vi "Dispatch Shutdown.vi"(8 "error in (no error)":errorcluster, 11 "Dispatcher in":refnum<class "Dispatcher Thread.lvclass">) -> (0 "error out":errorcluster, 3 "Dispatcher out":refnum<class "Dispatcher Thread.lvclass">)   [LabVIEW 2021, in "DSF Core.lvlib" / "Dispatcher Thread.lvclass"]
uses:
  Dispatcher Thread.lvclass
  C:/dev/git/custom-devices/niveristand-data-sharing-framework-custom-device/Source/Core/Classes/Thread/Thread.lvclass
  Dispatcher Thread.lvclass/Dispatcher Thread.ctl
  Interface/Dispatcher/Response Data.ctl
  Interface/Dispatcher/Response.ctl
  Interface/Dispatcher/Parameters.ctl
  Thread.lvclass/Thread.ctl
  <vilib>/NI/Memory Manager/Classes/Pointer/Pointer.lvclass/Pointer.ctl
  <vilib>/NI/Memory Manager/Classes/Pointer/Write Bool.vi
  <vilib>/NI/Memory Manager/Classes/Pointer/Write (No Check).vi
  <vilib>/NI/Memory Manager/Classes/Pointer/Write (No Check) Bool.vi
  <vilib>/NI/Memory Manager/Classes/Pointer/Check Move.vi
  <vilib>/NI/Memory Manager/Classes/Pointer/Get Address.vi
  <vilib>/NI/Memory Manager/Classes/Pointer/Check Null Pointer.vi
  <vilib>/NI/Memory Manager/Classes/Pointer/Check Count.vi
  <vilib>/NI/Memory Manager/Classes/Pointer/Check Bounds (Power of 2).vi
  <vilib>/NI/Memory Manager/Classes/Pointer/Errors.vi
  <vilib>/NI/Memory Manager/Classes/Pointer/Null Pointer.vi
  <vilib>/NI/Memory Manager/Classes/Pointer/Is Null.vi
  <vilib>/NI/Memory Manager/Classes/Pointer/Get Size.vi
  <vilib>/NI/Memory Manager/Classes/Pointer/Out of Bounds.vi
  <vilib>/NI/Memory Manager/Classes/Pointer/Check Bounds.vi
  <vilib>/NI/Memory Manager/Classes/Pointer/Create Error.vi
  <vilib>/NI/Memory Manager/VIs/Write String to Source.vi
  <vilib>/NI/Memory Manager/Classes/Pointer/Write Pointer Size to Error.vi
  <vilib>/NI/Memory Manager/VIs/Write Numeric to Source.vi
  <vilib>/NI/Memory Manager/VIs/Write Numeric Scalar to Source (Base10 U64).vi
  <vilib>/NI/Memory Manager/Classes/Pointer/Check Bounds (Pointer).vi
  <vilib>/NI/Memory Manager/Classes/Pointer/Check Bounds (Buffer).vi
  <vilib>/NI/Memory Manager/VIs/New Error Cluster.vi
  <vilib>/NI/Memory Manager/VIs/New Error Cluster (512B).vi
  <vilib>/NI/Memory Manager/VIs/Set Error Status.vi
  <vilib>/NI/Memory Manager/VIs/Set Error Code.vi
  <vilib>/NI/Memory Manager/VIs/Set Error Source.vi
  <vilib>/NI/Memory Manager/Constants/Constants.vi
  <vilib>/NI/Memory Manager/Constants/Library Name.vi
  <vilib>/NI/Memory Manager/Classes/Pointer/Pointer Error Info.vi
  <vilib>/NI/Memory Manager/Constants/Pointer Class Name.vi
  <vilib>/NI/Memory Manager/Classes/Pointer/Buffer Underflow.vi
  Interface/Dispatcher/Write Dispatcher Response.vi
  Interface/Plugin/Plugin Interface.lvclass
  Thread.lvclass
  Interface/Dispatcher/Dispatcher Interface.lvclass
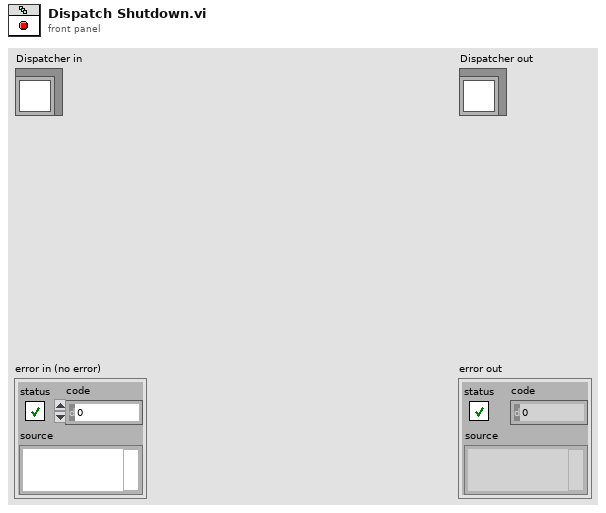
[diagram p1: front panel]
types:
  T1 = typedef "DSF Core.lvlib/Dispatcher Thread.lvclass/Plugin Settings.ctl" = cluster{"Transfer Group threads":i32[], "Plugin Thread Interfaces":refnum<class "Plugin Interface.lvclass">[]}
  T2 = typedef "DSF Core.lvlib/Dispatcher Interface.lvclass/Response Data.ctl" = cluster{"Response":T3, "Parameters":T4}
  T3 = typedef "DSF Core.lvlib/Dispatcher Interface.lvclass/Response.ctl" = enum8{"General Ack", "Error", "Shutting Down"}
  T4 = typedef "DSF Core.lvlib/Dispatcher Interface.lvclass/Parameters.ctl" = cluster{"arg1":u64, "arg2":u64}
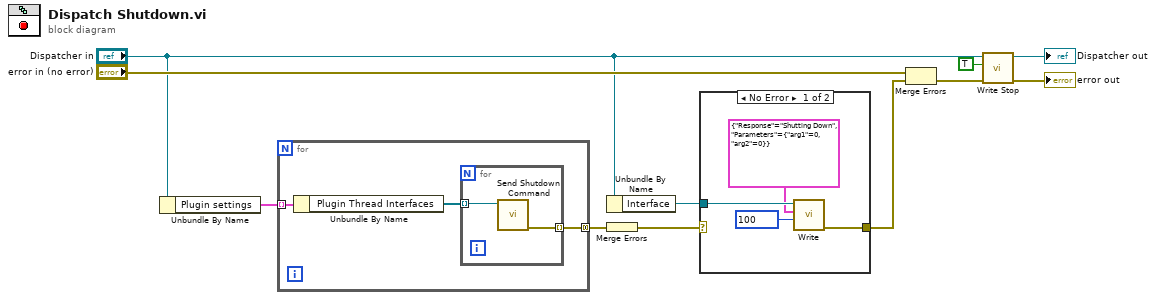
[diagram p0: block diagram]
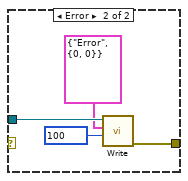
[diagram p2: hidden frame]
diagram:
  n1 = Unbundle By Name("Dispatcher in") -> ("Plugin settings"=w11:T1[])
  n2 = for {
    tunnel: w11 -> [w14] mode=indexing
    tunnel: [w12] -> w10 mode=concatenating
    n3 = Unbundle By Name(w14) -> ("Plugin Thread Interfaces"=w13:refnum<class "Plugin Interface.lvclass">[])
    n4 = for {
      tunnel: w13 -> [w16] mode=indexing
      tunnel: [w15] -> w12 mode=indexing
      n5 = call "Send Shutdown Command.vi"("Plugin Interface in"=w16) -> ("error out"=w15:errorcluster)  [unwired: 9 in, 1 out]
    }
  }
  n6 = Unbundle By Name("Dispatcher in") -> ("Interface"=w3:refnum<class "Dispatcher Interface.lvclass">)
  n7 = Merge Errors(w10) -> (w6:errorcluster)
  n8 = case shown="No Error" w6 {
    tunnel: [w19 w23] -> w5
    tunnel: w3 -> [w18 w22]
    frame No Error {
      n9 = call-poly <vilib>:"Write.vi"("timeout in ms (0)"=100, "response"=T2 {"Response"=enum."Shutting Down", "Parameters"={"arg1"=0, "arg2"=0}}, "Dispatcher Interface in"=w18) -> ("error out"=w19:errorcluster)  [unwired: 7 in, 1 out]
    }
    frame Error {
      n10 = call-poly <vilib>:"Write.vi"("timeout in ms (0)"=100, "response"=T2 {"Response"=enum."Error", "Parameters"={"arg1"=0, "arg2"=0}}, "Dispatcher Interface in"=w22) -> ("error out"=w23:errorcluster)  [unwired: 7 in, 1 out]
    }
  }
  n11 = Merge Errors("error in (no error)", w5) -> (w4:errorcluster)
  n12 = call "Write Stop.vi"("error in (no error)"=w4, "stop"=TRUE, "Thread in"="Dispatcher in") -> ("error out"=→"error out":errorcluster, "Thread out"=→"Dispatcher out":refnum<class "Dispatcher Thread.lvclass">)  [unwired: 7 in]
